vi "TestPlan - Device Mapping.vi"(7 "file path":path, 8 "error in":errorcluster, 11 "Test Type":T2 items=["Please Select", "Triaxial Shear", "Triaxial UU", "Shearbox", "Permeability", "Consolidation (Stepped Loading)/Swelling", "Saturation (Incremental)", "User Defined", "UCT", "Isotropic Consolidation", "Swelling Pressure"]) -> (0 "error out":errorcluster, 2 "Device Name":string[](array[string]), 3 "Key Name":string[](array[string]))   [LabVIEW 2019]
uses:
  Controls/Station - Tab Test Type.ctl
  Controls/Station - Test Type.ctl
  Controls/Station-state.ctl
  Controls/Station - Data Structure.ctl
  Controls/eFGV States.ctl
  Controls/Global - Device.vi
  Controls/Global - Channel.vi
  Controls/Global - Unit.vi
  <vilib>/Utility/miscctls.llb/LVRowAndColumnTypeDef.ctl
panel:
  out "ID":string
  in  "Refresh Button":bool
  out "Main Tab":enum32{"Blank", "Edit"}(tab)
  out "Sub Tab":T1
  out "Unit PPT Triaxial Shear":string caption="Cell Pressure Transducer"
  out "Unit Disp Triaxial Shear":string caption="Cell Pressure Transducer"
  out "Unit LT Triaxial Shear":string caption="Cell Pressure Transducer"
  out "Unit VC Triaxial Shear":string caption="Cell Pressure Transducer"
  out "Unit BPT Triaxial Shear":string caption="Cell Pressure Transducer"
  out "Unit CPT Triaxial Shear":string caption="Cell Pressure Transducer"
  in  "VLC Triaxial Shear":u16(ring) caption="Vertical Load Control" items=["Please Select"]
  in  "BPC Triaxial Shear":u16(ring) caption="Back Pressure Control" items=["Please Select"]
  out "Disp Triaxial Shear":sgl caption="Dispalcement" format="%.5f"
  out "PPT Triaxial Shear":sgl caption="Pore Pressure Transduser" format="%.5f"
  out "LT Triaxial Shear":sgl caption="Load Tranduser" format="%.5f"
  out "BPT Triaxial Shear":sgl caption="Back Pressure Transducer" format="%.5f"
  out "VC Triaxial Shear":sgl caption="Volume Change" format="%.5f"
  out "CPT Triaxial Shear":sgl caption="Cell Pressure Transducer" format="%.5f"
  in  "CPC Triaxial Shear":u16(ring) caption="Cell Pressure Control" items=["Please Select"]
  in  "VLC Triaxial UU":u16(ring) caption="Vertical Load Control" items=["Please Select"]
  out "CPT Triaxial UU":sgl caption="Cell Pressure" format="%.5f"
  out "VLT Triaxial UU":sgl caption="Vertical Load" format="%.5f"
  out "PPT Triaxial UU":sgl caption="Pore Pressure" format="%.5f"
  out "Disp Triaxial UU":sgl caption="Displacement" format="%.5f"
  in  "CPC Triaxial UU":u16(ring) caption="Cell Pressure Control" items=["Please Select"]
  out "Unit CPT Triaxial UU":string caption="Cell Pressure Transducer"
  out "Unit VLT Triaxial UU":string caption="Cell Pressure Transducer"
  out "Unit Disp Triaxial UU":string caption="Cell Pressure Transducer"
  out "Unit PPT Triaxial UU":string caption="Cell Pressure Transducer"
  in  "HLC Shearbox":u16(ring) caption="Horinzontal Load Control" items=["Please Select"]
  out "LT Shearbox":sgl caption="Vertical Load Tranducer" format="%.5f"
  out "Disp Shearbox":sgl caption="Vertical Dispalcement" format="%.5f"
  out "H Dis Shearbox":sgl caption="Horizontal Dispalcement" format="%.5f"
  out "HLT Shearbox":sgl caption="Horinzontal Load Tranducer" format="%.5f"
  in  "VLC Shearbox":u16(ring) caption="Vertical Load Control" items=["Please Select"]
  out "Unit LT Shearbox":string caption="Cell Pressure Transducer"
  out "Unit Disp Shearbox":string caption="Cell Pressure Transducer"
  out "Unit HLT Shearbox":string caption="Cell Pressure Transducer"
  out "Unit H Dis Shearbox":string caption="Cell Pressure Transducer"
  in  "BPC2 Permeability":u16(ring) caption="Back Pressure 2 Control" items=["Please Select"]
  in  "BPC Permeability":u16(ring) caption="Back Pressure Control" items=["Please Select"]
  out "BPT2 Permeability":sgl caption="Back Pressure 2" format="%.5f"
  out "PPT Permeability":sgl caption="Pore Pressure" format="%.5f"
  out "OVC Permeability":sgl caption="Outlet Volume Change" format="%.5f"
  out "BPT Permeability":sgl caption="Back Pressure" format="%.5f"
  out "IVC Permeability":sgl caption="Inlet Volume Change" format="%.5f"
  out "CPT Permeability":sgl caption="Cell Pressure" format="%.5f"
  in  "CPC Permeability":u16(ring) caption="Cell Pressure Control" items=["Please Select"]
  out "Unit CPT Permeability":string caption="Cell Pressure Transducer"
  out "Unit BPT Permeability":string caption="Cell Pressure Transducer"
  out "Unit IVC Permeability":string caption="Cell Pressure Transducer"
  out "Unit BPT2 Permeability":string caption="Cell Pressure Transducer"
  out "Unit OVC Permeability":string caption="Cell Pressure Transducer"
  out "Unit PPT Permeability":string caption="Cell Pressure Transducer"
  out "Disp Consolidation":sgl caption="Dispalcement"
  out "LT Consolidation":sgl caption="Load Tranducer"
  in  "VLC Consolidation":u16(ring) caption="Vertical Load  Control" items=["Please Select"]
  out "Unit LT Consolidation":string caption="Cell Pressure Transducer"
  out "Unit Disp Consolidation":string caption="Cell Pressure Transducer"
  out "CPT Saturation":sgl caption="Cell Pressure Transducer" format="%.5f"
  out "VC Saturation":sgl caption="Volume Change" format="%.5f"
  out "BPT Saturation":sgl caption="Back Pressure Transducer" format="%.5f"
  out "PPT Saturation":sgl caption="Pore pressure Tranduser" format="%.5f"
  in  "CPC Saturation":u16(ring) caption="Cell Pressure Control" items=["Please Select"]
  in  "BPC Saturation":u16(ring) caption="Back Pressure Control" items=["Please Select"]
  out "Unit CPT Saturation":string caption="Cell Pressure Transducer"
  out "Unit BPT Saturation":string caption="Cell Pressure Transducer"
  out "Unit VC Saturation":string caption="Cell Pressure Transducer"
  out "Unit PPT Saturation":string caption="Cell Pressure Transducer"
  out "HD User Defined":sgl caption="Horizontal Displacement"
  out "HL User Defined":sgl caption="Horizontal Load"
  out "VD User Defined":sgl caption="Vertical Displacement"
  out "VC2 User Defined":sgl caption="Volume Change 2"
  out "VC1 User Defined":sgl caption="Volume Change 1"
  out "VL User Defined":sgl caption="Vertical Load"
  out "BPT2 User Defined":sgl caption="Back Pressure 2"
  out "PWP User Defined":sgl caption="Pore Water Pressure"
  out "BPT User Defined":sgl caption="Back Pressure"
  out "CPT User Defined":sgl caption="Cell Pressure"
  in  "HLC User Defined":u16(ring) caption="Horizontal Load Control" items=["Please Select"]
  in  "VLC User Defined":u16(ring) caption="Vertical Load Control" items=["Please Select"]
  in  "BPC2 User Defined":u16(ring) caption="Back Pressure 2 Control" items=["Please Select"]
  in  "BPC User Defined":u16(ring) caption="Back Pressure Control" items=["Please Select"]
  in  "CPC User Defined":u16(ring) caption="Cell Pressure Control" items=["Please Select"]
  out "Unit CPT User Defined":string caption="Cell Pressure Transducer"
  out "Unit BPT User Defined":string caption="Cell Pressure Transducer"
  out "Unit VC1 User Defined":string caption="Cell Pressure Transducer"
  out "Unit PWP User Defined":string caption="Cell Pressure Transducer"
  out "Unit BPT2 User Defined":string caption="Cell Pressure Transducer"
  out "Unit VC2 User Defined":string caption="Cell Pressure Transducer"
  out "Unit HD User Defined":string caption="Cell Pressure Transducer"
  out "Unit HL User Defined":string caption="Cell Pressure Transducer"
  out "Unit VD User Defined":string caption="Cell Pressure Transducer"
  out "Unit VL User Defined":string caption="Cell Pressure Transducer"
  in  "save edit":bool
  in  "DELETE STATION":bool
  in  "Table":i32(listbox)
  in  "OK":bool
  in  "CREATE NEW STATION":bool
  # "Live Reading"
  # "Live Reading"
  # "Live Reading"
  # "Live Reading"
  # "Live Reading"
  # "Live Reading"
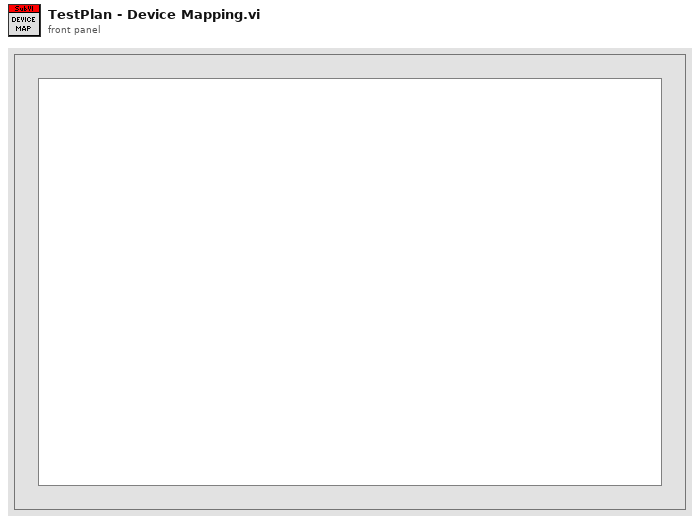
[diagram p1: front panel]
types:
  T1 = typedef "Station - Tab Test Type.ctl" = enum32{"Please Select", "Triaxial Shear", "Triaxial UU", "Shearbox", "Permeability", "Consolidation", "Saturation", "User Defined", "UCT", "Isotropic Consolidation"}
  T2 = typedef "Station - Test Type.ctl" = u16
  T3 = typedef "Station-state.ctl" = enum16{"Init", "Read Config", "Idle", "Delete", "Upload", "save edit", "update stationid", "Close", "Read sensor", "Exit"}
  T4 = typedef "eFGV States.ctl" = enum16{"Init", "Read", "Write", "Exit"}
  T5 = typedef "Station - Data Structure.ctl" = cluster{"Table station":string[][], "Station Name":string, "EditRow":i32, "Station ID":string}
  T6 = cluster{"TestPlan Section":string, "Key Value":string[]}[]
  T7 = cluster{"TestPlan Section":string, "Key Value":string[]}
  T8 = typedef "UDP - Event.ctl" = u16
  T9 = typedef "UDP - Status.ctl" = u16
  T10 = cluster{"Channels":cluster{"Ch1":sgl, "Ch2":sgl, "Ch3":sgl, "Ch4":sgl, "Ch5":sgl, "Ch6":sgl, "Ch7":sgl, "Ch8":sgl, "Ch9":sgl, "Ch10":sgl, "Ch11":sgl, "Ch12":sgl, "Ch13":sgl, "Ch14":sgl, "Ch15":sgl, "Ch16":sgl}, "Event":T8, "Status":T9, "IP":string}[]
  T11 = cluster{"Name":string[], "Unit":string[], "Decimal Point":u8[], "Ch Log":u8[], "H Alarm":u8[], "L Alarm":u8[], "H Limit":sgl[], "L Limit":sgl[], "Filter":u8[], "Gain":u8[], "Calib Type":u32[]}[]
  T12 = cluster{"Channels":cluster{"Ch1":sgl, "Ch2":sgl, "Ch3":sgl, "Ch4":sgl, "Ch5":sgl, "Ch6":sgl, "Ch7":sgl, "Ch8":sgl, "Ch9":sgl, "Ch10":sgl, "Ch11":sgl, "Ch12":sgl, "Ch13":sgl, "Ch14":sgl, "Ch15":sgl, "Ch16":sgl}, "Event":T8, "Status":T9, "IP":string}
  T13 = cluster{"Name":string[], "Unit":string[], "Decimal Point":u8[], "Ch Log":u8[], "H Alarm":u8[], "L Alarm":u8[], "H Limit":sgl[], "L Limit":sgl[], "Filter":u8[], "Gain":u8[], "Calib Type":u32[]}
  T14 = cluster{"Station Name":string, "Key Value":string[], "Key Names":string[]}[]
  T15 = cluster{"Station Name":string, "Key Value":string[], "Key Names":string[]}
  T16 = typedef "LVRowAndColumnTypeDef.ctl" = cluster{"Row":i32, "Column":i32}
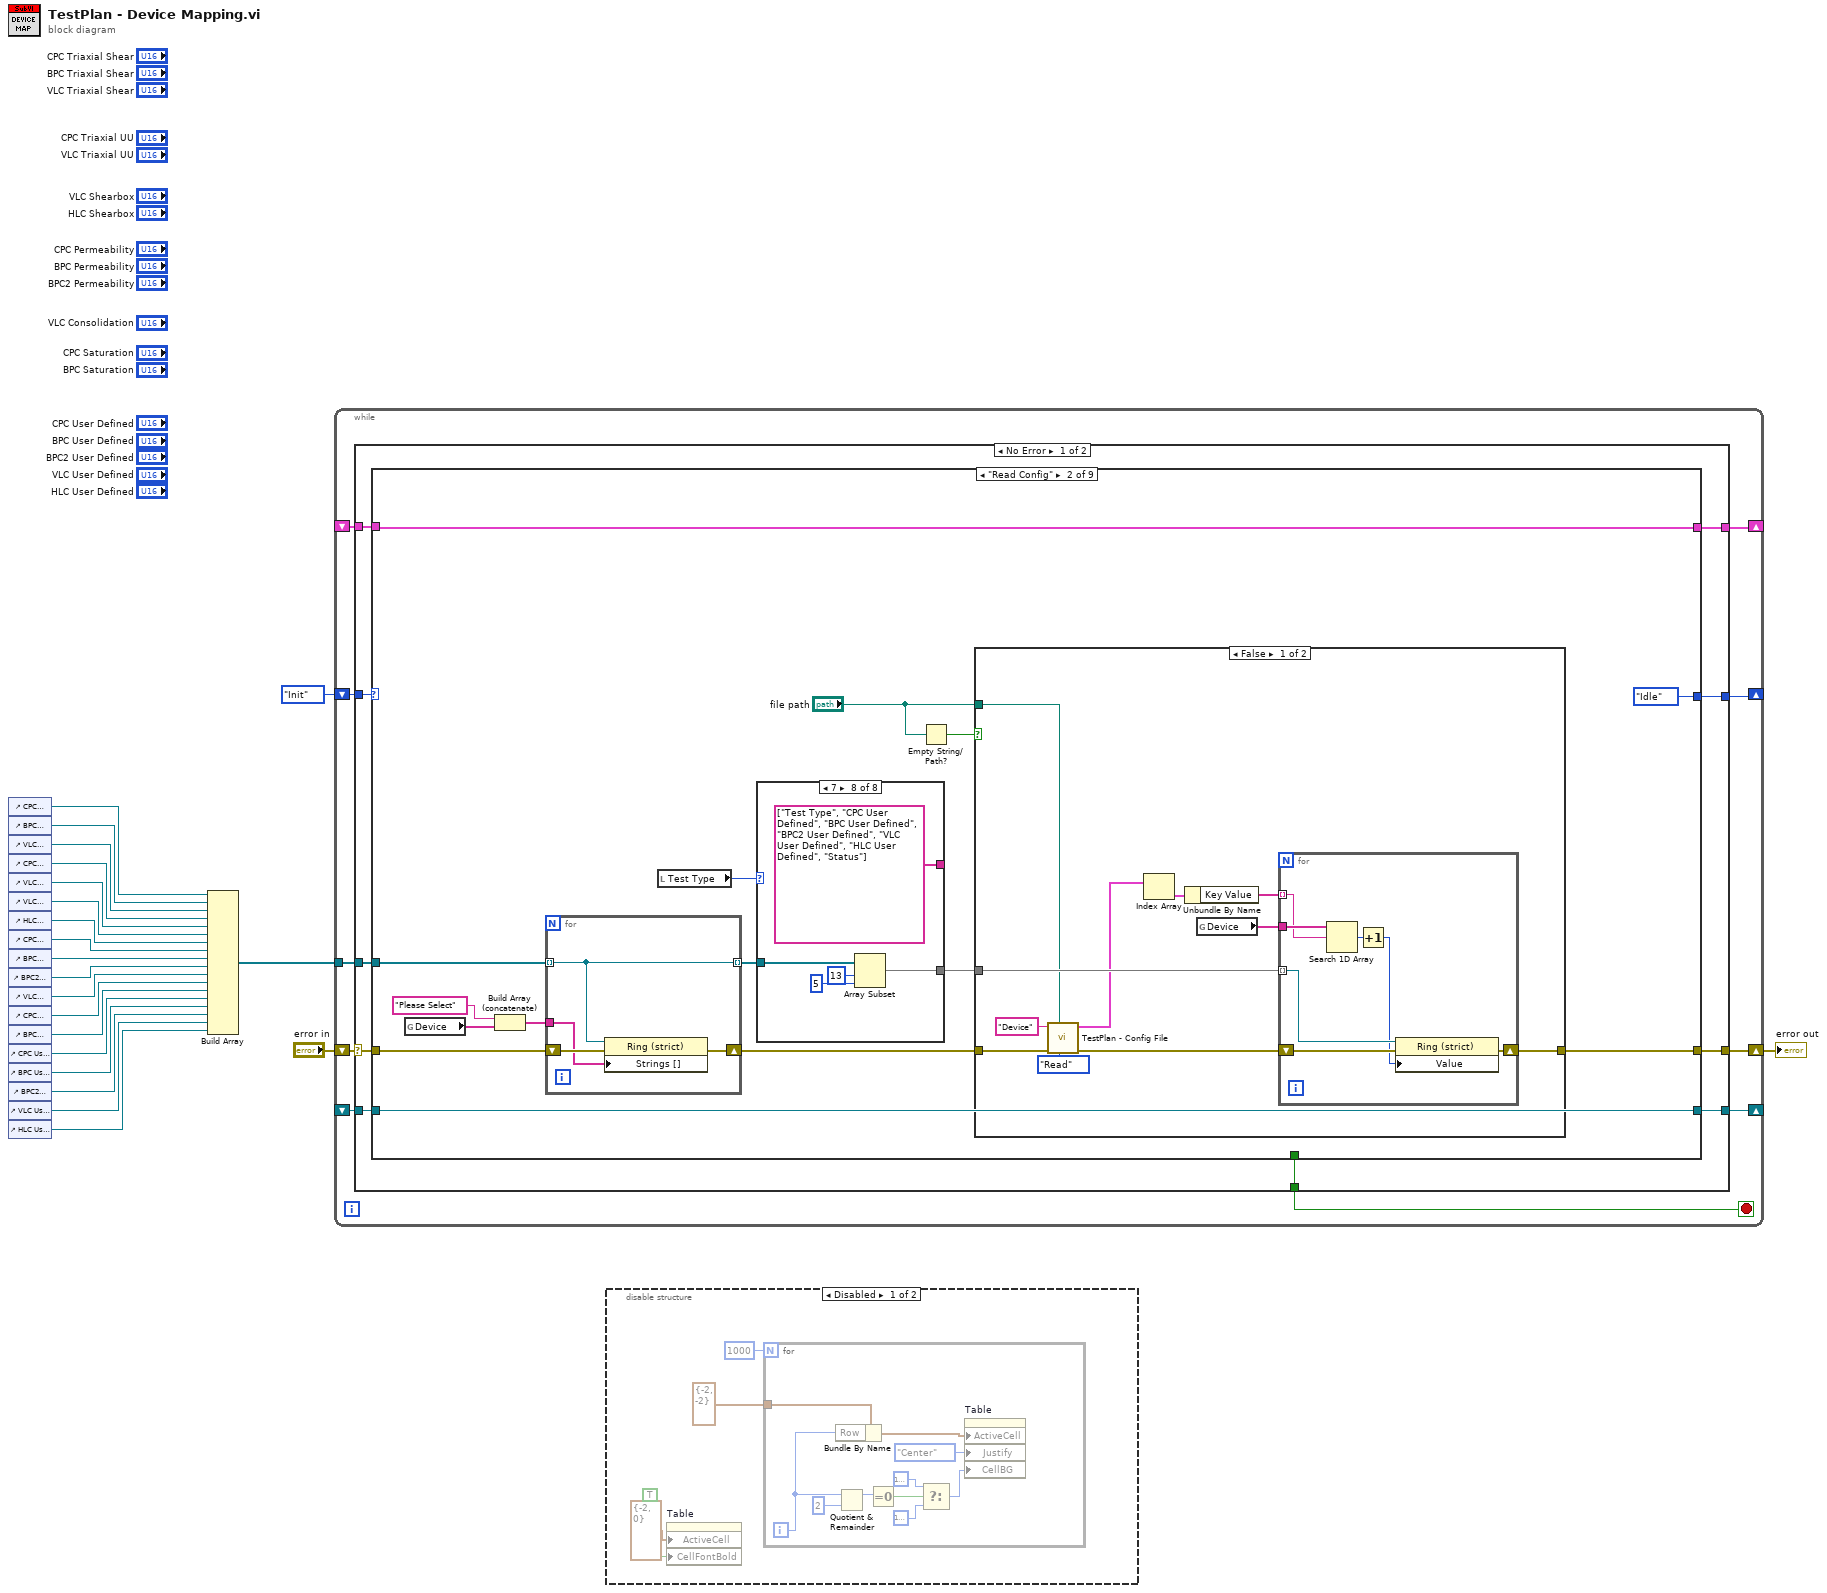
[diagram p0: block diagram]
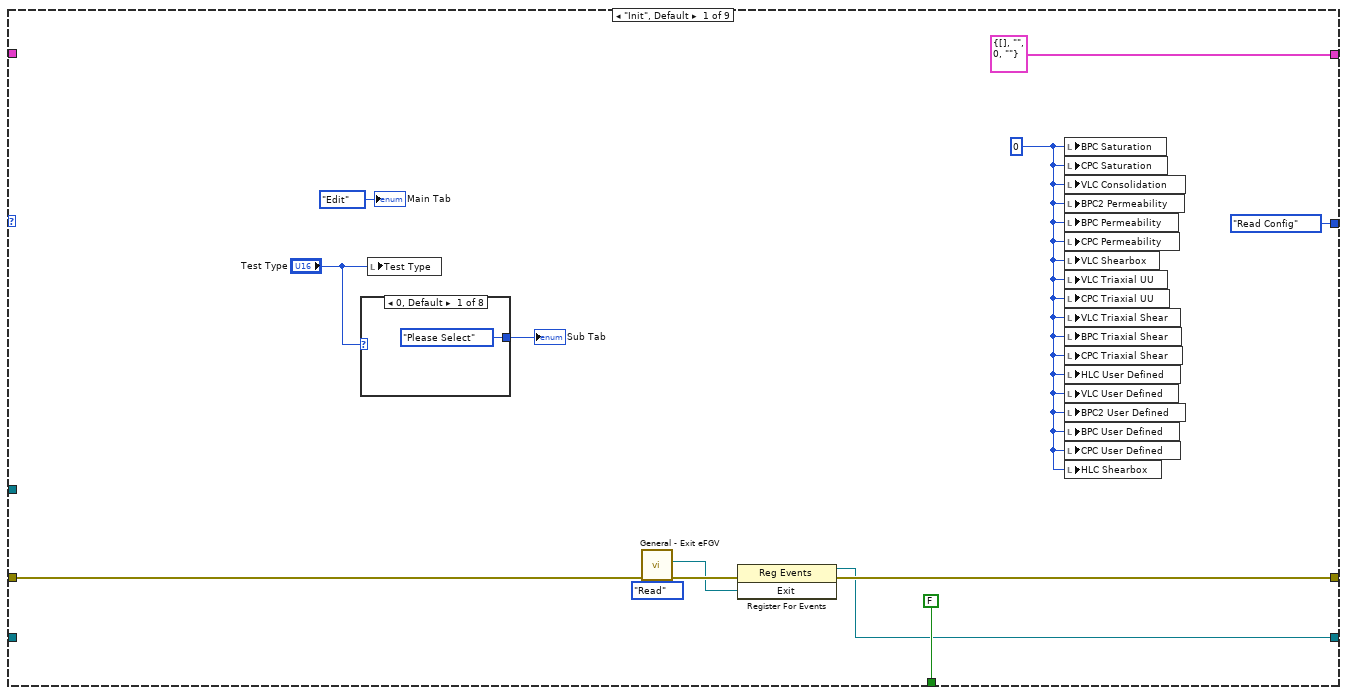
[diagram p2: hidden frame]
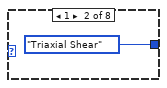
[diagram p3: hidden frame]
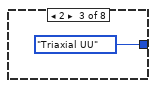
[diagram p4: hidden frame]
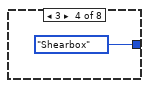
[diagram p5: hidden frame]
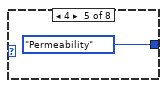
[diagram p6: hidden frame]
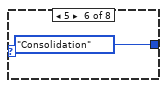
[diagram p7: hidden frame]
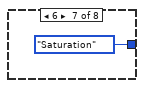
[diagram p8: hidden frame]
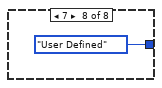
[diagram p9: hidden frame]
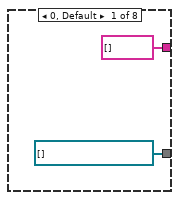
[diagram p11: hidden frame]
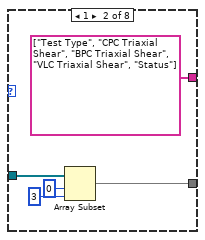
[diagram p12: hidden frame]
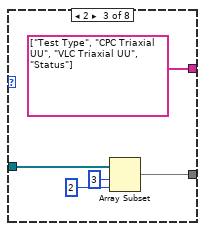
[diagram p13: hidden frame]
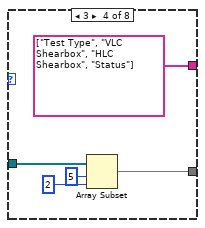
[diagram p14: hidden frame]
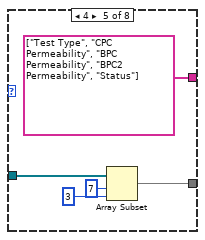
[diagram p15: hidden frame]
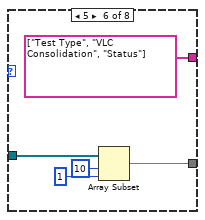
[diagram p16: hidden frame]
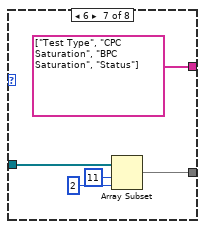
[diagram p17: hidden frame]
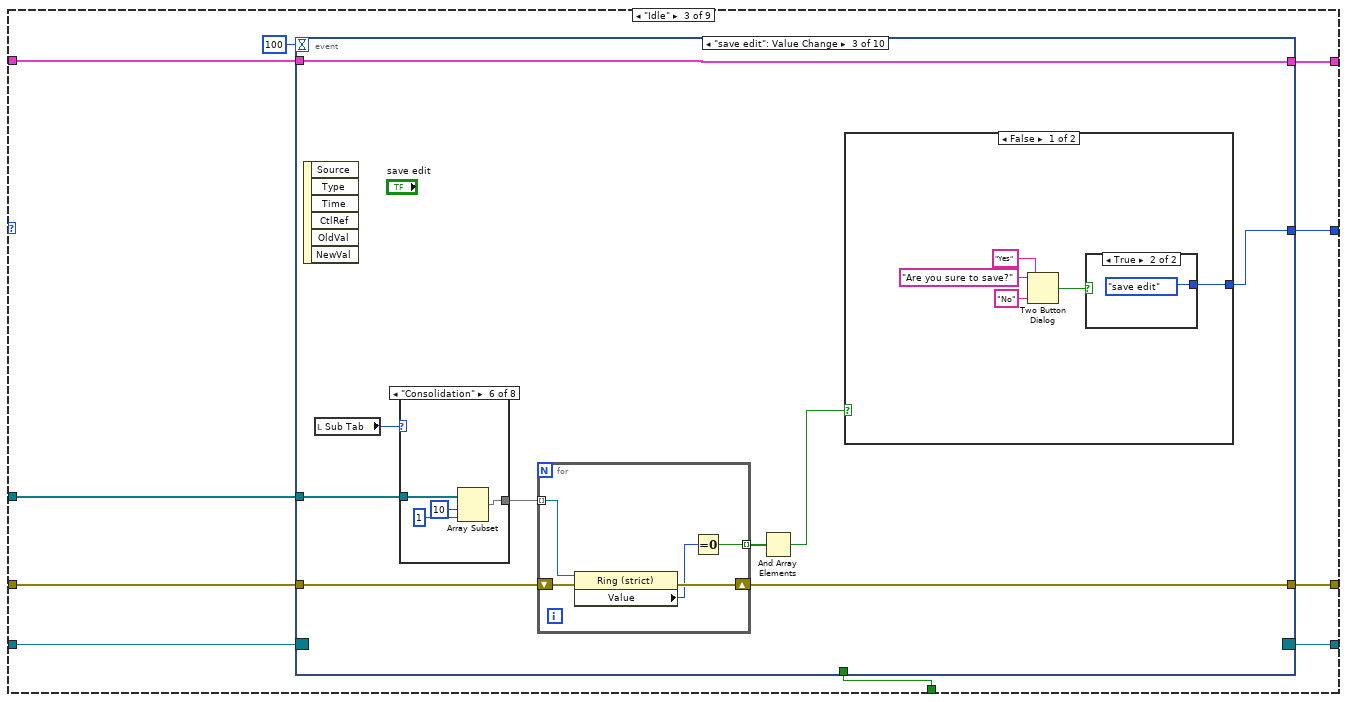
[diagram p18: hidden frame]
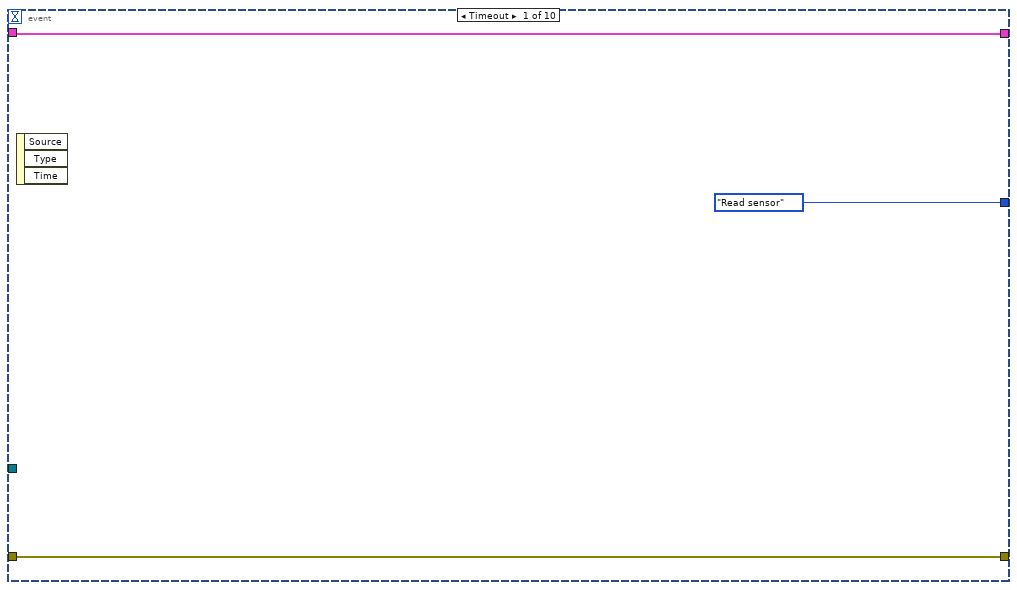
[diagram p19: hidden frame]
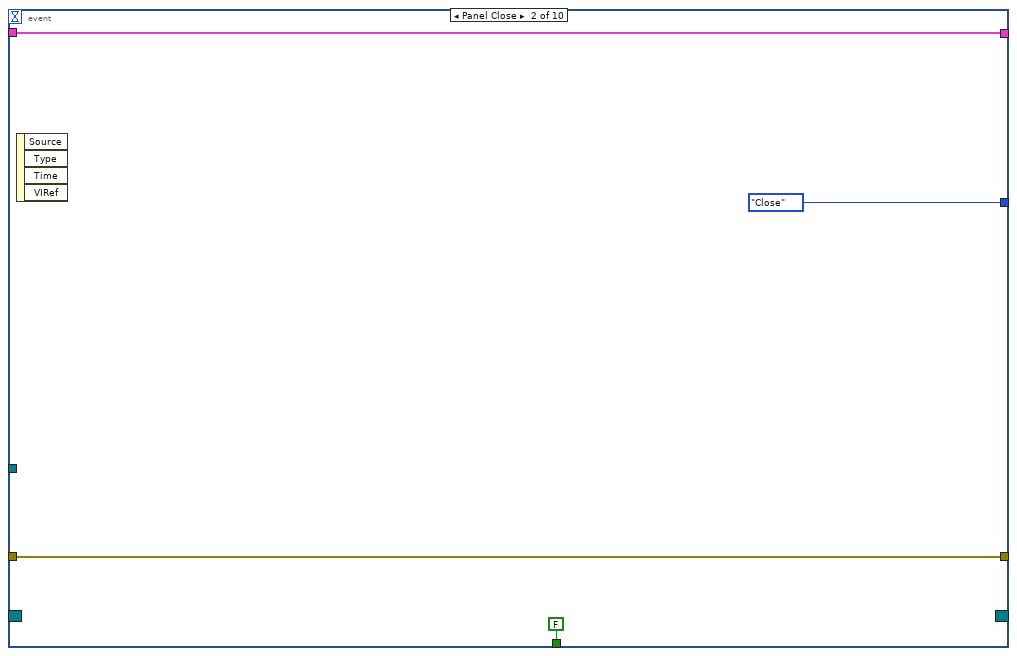
[diagram p20: hidden frame]
diagram:
  n1 = control-ref of="CPC Triaxial Shear"() -> (w19:refnum<vi>)
  n2 = control-ref of="BPC Triaxial Shear"() -> (w18:refnum<vi>)
  n3 = control-ref of="VLC Triaxial Shear"() -> (w17:refnum<vi>)
  n4 = control-ref of="CPC Triaxial UU"() -> (w16:refnum<vi>)
  n5 = control-ref of="VLC Triaxial UU"() -> (w15:refnum<vi>)
  n6 = control-ref of="VLC Shearbox"() -> (w14:refnum<vi>)
  n7 = control-ref of="HLC Shearbox"() -> (w13:refnum<vi>)
  n8 = control-ref of="CPC Permeability"() -> (w12:refnum<vi>)
  n9 = control-ref of="BPC Permeability"() -> (w11:refnum<vi>)
  n10 = control-ref of="BPC2 Permeability"() -> (w10:refnum<vi>)
  n11 = control-ref of="VLC Consolidation"() -> (w9:refnum<vi>)
  n12 = control-ref of="CPC Saturation"() -> (w8:refnum<vi>)
  n13 = control-ref of="BPC Saturation"() -> (w7:refnum<vi>)
  n14 = control-ref of="CPC User Defined"() -> (w6:refnum<vi>)
  n15 = control-ref of="BPC User Defined"() -> (w5:refnum<vi>)
  n16 = control-ref of="BPC2 User Defined"() -> (w4:refnum<vi>)
  n17 = control-ref of="VLC User Defined"() -> (w3:refnum<vi>)
  n18 = control-ref of="HLC User Defined"() -> (w2:refnum<vi>)
  n19 = Build Array(w19, w18, w17, w16, w15, w14, w13, w12, w11, w10, w9, w8, w7, w6, w5, w4, w3, w2) -> (w1:refnum<vi>[])
  n20 = while {
    shift-right: [w31] -> w21
    shift-left: "error in" -> [w32]
    shift-right: [w29] -> _
    shift-left: Station-state."Init" -> [w30]
    shift-right: [w27] -> _
    shift-left: _ -> [w26]
    shift-right: [w25] -> _
    shift-left: _ -> [w24]
    tunnel: w1 -> [w23]
    stop <- w28 stop-if-true
    n21 = case shown="No Error" w32 {
      selector: w32 -> [w41 w699]
      tunnel: [w40 w700] -> w31
      tunnel: w30 -> [w42 _]
      tunnel: [w39 Station-state."Idle"] -> w29
      tunnel: [w38 _] -> w28
      tunnel: [w37 w709] -> w27
      tunnel: w26 -> [w36 w709]
      tunnel: [w35 w707] -> w25
      tunnel: w24 -> [w34 w707]
      tunnel: w23 -> [w33 _]
      frame No Error {
        n22 = case shown="\"Read Config\"" w42 {
          tunnel: w41 -> [w43 w74 w148 w274 w553 w585 w641 w691 w692]
          tunnel: [w52 w70 w147 w273 w554 w570 w637 w688 w693] -> w40
          tunnel: [Station-state."Read Config" Station-state."Idle" w145 Station-state."Idle" Station-state."Read Config" Station-state."Idle" Station-state."Exit" Station-state."Idle" Station-state."Exit"] -> w39
          tunnel: [FALSE _ w146 _ _ _ _ _ TRUE] -> w38
          tunnel: [T5 {"Table station"=[], "Station Name"="", "EditRow"=0, "Station ID"=""} w71 w143 w279 w558 w562 w638 w690 w698] -> w37
          tunnel: w36 -> [_ w71 w144 w279 w558 w561 w638 w690 w698]
          tunnel: [w50 w77 w141 w278 w557 w590 w643 w686 w697] -> w35
          tunnel: w34 -> [_ w77 w142 w278 w557 w590 w643 w686 w697]
          tunnel: w33 -> [_ w73 w139 w271 _ w567 w640 _ _]
          frame "Init", Default {
            w46 = 0
            n23 = case shown="0, Default" "Test Type" {
              tunnel: [Station_-_Tab_Test_Type."Please Select" ("Sub Tab") Station_-_Tab_Test_Type."Triaxial Shear" ("Sub Tab") Station_-_Tab_Test_Type."Triaxial UU" ("Sub Tab") Station_-_Tab_Test_Type."Shearbox" ("Sub Tab") Station_-_Tab_Test_Type."Permeability" ("Sub Tab") Station_-_Tab_Test_Type."Consolidation" ("Sub Tab") Station_-_Tab_Test_Type."Saturation" ("Sub Tab") Station_-_Tab_Test_Type."User Defined" ("Sub Tab")] -> w44
              frame 0, Default {
              }
              frame 1 {
              }
              frame 2 {
              }
              frame 3 {
              }
              frame 4 {
              }
              frame 5 {
              }
              frame 6 {
              }
              frame 7 {
              }
            }
            "Sub Tab" <- w44
            n24 = local write "Test Type"("Test Type") -> ()
            n25 = call "General - Exit eFGV.vi"("eFGV States"=eFGV_States."Read", "error in (no error)"=w43) -> ("error out"=w53:errorcluster, "Exit"=w51:refnum<user-event>)  [unwired: 7 in, 1 out]
            n26 = register-events(error in=w53, w51) -> (reference out=w50:refnum<event-registration>, error out=w52:errorcluster)  [unwired: 1 in]
            n27 = local write "BPC Saturation"(w46) -> ()
            n28 = local write "CPC Saturation"(w46) -> ()
            n29 = local write "VLC Consolidation"(w46) -> ()
            n30 = local write "BPC2 Permeability"(w46) -> ()
            n31 = local write "BPC Permeability"(w46) -> ()
            n32 = local write "CPC Permeability"(w46) -> ()
            n33 = local write "VLC Shearbox"(w46) -> ()
            n34 = local write "VLC Triaxial UU"(w46) -> ()
            n35 = local write "CPC Triaxial UU"(w46) -> ()
            n36 = local write "VLC Triaxial Shear"(w46) -> ()
            n37 = local write "BPC Triaxial Shear"(w46) -> ()
            n38 = local write "CPC Triaxial Shear"(w46) -> ()
            n39 = local write "HLC User Defined"(w46) -> ()
            n40 = local write "VLC User Defined"(w46) -> ()
            n41 = local write "BPC2 User Defined"(w46) -> ()
            n42 = local write "BPC User Defined"(w46) -> ()
            n43 = local write "CPC User Defined"(w46) -> ()
            n44 = local write "HLC Shearbox"(w46) -> ()
            "Main Tab" <- enum32{"Blank", "Edit"}."Edit" ("Main Tab")
          }
          frame "Read Config" {
            n45 = global read "Global - Device.vi" "Device"() -> (w72:string[])
            n46 = Build Array (concatenate)("Please Select", w72) -> (w75:string[])
            n47 = for {
              shift-right: [w137] -> w66
              shift-left: w74 -> [w138]
              tunnel: w73 -> [w135] mode=indexing
              tunnel: w75 -> [w136]
              tunnel: [w135] -> w69 mode=indexing
              n48 = property class="Ring (strict)"(reference=w135, error in=w138, "Strings []"=w136) -> (error out=w137:errorcluster)  [unwired: 1 out]
            }
            n49 = local read "Test Type"() -> (w68:T2)
            n50 = case shown="7" w68 {
              tunnel: [string[] [] string[] ["Test Type", "CPC Triaxial Shear", "BPC Triaxial Shear", "VLC Triaxial Shear", "Status"] string[] ["Test Type", "CPC Triaxial UU", "VLC Triaxial UU", "Status"] string[] ["Test Type", "VLC Shearbox", "HLC Shearbox", "Status"] string[] ["Test Type", "CPC Permeability", "BPC Permeability", "BPC2 Permeability", "Status"] string[] ["Test Type", "VLC Consolidation", "Status"] string[] ["Test Type", "CPC Saturation", "BPC Saturation", "Status"] string[] ["Test Type", "CPC User Defined", "BPC User Defined", "BPC2 User Defined", "VLC User Defined", "HLC User Defined", "Status"]] -> _
              tunnel: w69 -> [_ w103 w106 w111 w116 w121 w126 w131]
              tunnel: [refnum<vi>[] [] w100 w105 w110 w115 w120 w125 w130] -> w67
              frame 0, Default {
              }
              frame 1 {
                n51 = Array Subset(array=w103, index=0, length=3) -> (w100:refnum<vi>[])
              }
              frame 2 {
                n52 = Array Subset(array=w106, index=3, length=2) -> (w105:refnum<vi>[])
              }
              frame 3 {
                n53 = Array Subset(array=w111, index=5, length=2) -> (w110:refnum<vi>[])
              }
              frame 4 {
                n54 = Array Subset(array=w116, index=7, length=3) -> (w115:refnum<vi>[])
              }
              frame 5 {
                n55 = Array Subset(array=w121, index=10, length=1) -> (w120:refnum<vi>[])
              }
              frame 6 {
                n56 = Array Subset(array=w126, index=11, length=2) -> (w125:refnum<vi>[])
              }
              frame 7 {
                n57 = Array Subset(array=w131, index=13, length=5) -> (w130:refnum<vi>[])
              }
            }
            n58 = Empty String/Path?(string/path="file path") -> (empty?=w64:bool)
            n59 = case shown="False" w64 {
              tunnel: [w88 w97] -> w70
              tunnel: w67 -> [w87 _]
              tunnel: w66 -> [w85 w97]
              tunnel: "file path" -> [w79 _]
              frame False {
                n60 = call "TestPlan - Config File.vi"("Action"=enum16{"Write", "Read", "Read All", "Remove"}."Read", "file path"=w79, "error in (no error)"=w85, "TestPlan Section"="Device") -> ("error out"=w84:errorcluster, "Value Out"=w83:T6)  [unwired: 5 in, 1 out]
                n61 = Index Array(array=w83) -> (element=w81:T7)  [unwired: 1 in]
                n62 = Unbundle By Name(w81) -> ("Key Value"=w80:string[])
                n63 = global read "Global - Device.vi" "Device"() -> (w89:string[])
                n64 = for {
                  tunnel: w80 -> [w95] mode=indexing
                  tunnel: w89 -> [w96]
                  shift-right: [w93] -> w88
                  shift-left: w84 -> [w94]
                  tunnel: w87 -> [w92] mode=indexing
                  n65 = Search 1D Array(1D array=w96, element=w95) -> (index of element=w91:i32)  [unwired: 1 in]
                  n66 = Increment(x=w91) -> (x+1=w90:i32)
                  n67 = property class="Ring (strict)"(reference=w92, error in=w94, "Value"=w90) -> (error out=w93:errorcluster)  [unwired: 1 out]
                }
              }
              frame True {
              }
            }
          }
          frame "Idle" {
            n68 = event shown="[2] \"save edit\": Value Change" {
              selector: w142 -> [_ _ _ _ _ _ _ _ _ _]
              dyn-events: [_ _ _ _ _ _ _ _ _ _] -> w141
              timeout: 100 -> [_ _ _ _ _ _ _ _ _ _]
              tunnel: w148 -> [w149 w155 w159 w209 w229 w232 w238 w247 w250 w252]
              tunnel: [w149 w155 w156 w209 w229 w232 w237 w247 w250 w253] -> w147
              tunnel: [_ FALSE _ _ _ _ _ _ FALSE _] -> w146
              tunnel: [Station-state."Read sensor" Station-state."Close" w163 Station-state."Idle" w225 Station-state."Read Config" w234 Station-state."Exit" Station-state."Close" w257] -> w145
              tunnel: w144 -> [w151 w154 w164 w211 w221 w231 w239 w246 w249 w254]
              tunnel: [w151 w154 w164 w211 w221 w231 w239 w246 w249 w255] -> w143
              tunnel: w139 -> [_ _ w162 _ _ _ _ _ _ _]
              event Timeout {
                n69 = event-data() -> ()  [unwired: 1 in, 3 out]
              }
              event Panel Close {
                n70 = event-data() -> ()  [unwired: 1 in, 4 out]
              }
              event "save edit": Value Change {
                n71 = event-data() -> ()  [unwired: 1 in, 6 out]
                n72 = local read "Sub Tab"() -> (w161:T1)
                n73 = case shown="\"Consolidation\"" w161 {
                  tunnel: w162 -> [_ w183 w185 w189 w193 w197 w201 w205]
                  tunnel: [_ w180 w184 w188 w192 w196 w200 w204] -> w160
                  frame "Please Select", Default {
                  }
                  frame "Triaxial Shear" {
                    n74 = Array Subset(array=w183, index=0, length=3) -> (w180:refnum<vi>[])
                  }
                  frame "Triaxial UU" {
                    n75 = Array Subset(array=w185, index=3, length=2) -> (w184:refnum<vi>[])
                  }
                  frame "Shearbox" {
                    n76 = Array Subset(array=w189, index=5, length=2) -> (w188:refnum<vi>[])
                  }
                  frame "Permeability" {
                    n77 = Array Subset(array=w193, index=7, length=3) -> (w192:refnum<vi>[])
                  }
                  frame "Consolidation" {
                    n78 = Array Subset(array=w197, index=10, length=1) -> (w196:refnum<vi>[])
                  }
                  frame "Saturation" {
                    n79 = Array Subset(array=w201, index=11, length=2) -> (w200:refnum<vi>[])
                  }
                  frame "User Defined" {
                    n80 = Array Subset(array=w205, index=13, length=5) -> (w204:refnum<vi>[])
                  }
                }
                n81 = for {
                  tunnel: w160 -> [w177] mode=indexing
                  shift-right: [w178] -> w156
                  shift-left: w159 -> [w179]
                  tunnel: [w175] -> w158 mode=indexing
                  n82 = property class="Ring (strict)"(reference=w177, error in=w179) -> (error out=w178:errorcluster, "Value"=w176:u16)  [unwired: 1 out]
                  n83 = Equal To 0?(x=w176) -> (x = 0?=w175:bool)
                }
                n84 = And Array Elements(Boolean array=w158) -> (logical AND=w157:bool)
                n85 = case shown="False" w157 {
                  tunnel: [w169 Station-state."Idle"] -> w163
                  frame False {
                    n86 = Two Button Dialog(message="Are you sure to save?", 1:"No" ("F button name (\"Cancel\")"), 2:"Yes" ("T button name (\"OK\")")) -> (T button?=w168:bool)
                    n87 = case shown="True" w168 {
                      tunnel: [Station-state."Idle" Station-state."save edit"] -> w169
                      frame False {
                      }
                      frame True {
                      }
                    }
                  }
                  frame True {
                    n88 = One Button Dialog(message="Please Select Device", button name ("OK")="OK") -> ()  [unwired: 1 out]
                  }
                }
              }
              event Value Change {
                n89 = event-data() -> ("NewVal"=w210:T2)  [unwired: 1 in, 5 out]
                n90 = case shown="0, Default" w210 {
                  tunnel: [Station_-_Tab_Test_Type."Please Select" ("Sub Tab") Station_-_Tab_Test_Type."Triaxial Shear" ("Sub Tab") Station_-_Tab_Test_Type."Triaxial UU" ("Sub Tab") Station_-_Tab_Test_Type."Shearbox" ("Sub Tab") Station_-_Tab_Test_Type."Permeability" ("Sub Tab") Station_-_Tab_Test_Type."Consolidation" ("Sub Tab") Station_-_Tab_Test_Type."Saturation" ("Sub Tab") Station_-_Tab_Test_Type."User Defined" ("Sub Tab")] -> w208
                  frame 0, Default {
                  }
                  frame 1 {
                  }
                  frame 2 {
                  }
                  frame 3 {
                  }
                  frame 4 {
                  }
                  frame 5 {
                  }
                  frame 6 {
                  }
                  frame 7 {
                  }
                }
                n91 = local write "Sub Tab"(w208) -> ()
              }
              event "DELETE STATION": Value Change {
                n92 = event-data() -> ()  [unwired: 1 in, 6 out]
                n93 = Two Button Dialog(message="Are you sure to delete?", 1:"No" ("F button name (\"Cancel\")"), 2:"Yes" ("T button name (\"OK\")")) -> (T button?=w222:bool)
                n94 = Select(t=Station-state."Delete", s=w222, f=Station-state."Idle") -> (s? t:f=w225:T3)
              }
              event "Refresh Button": Value Change {
                n95 = event-data() -> ()  [unwired: 1 in, 6 out]
              }
              event "CREATE NEW STATION": Value Change {
                n96 = event-data() -> ()  [unwired: 1 in, 6 out]
                n97 = disable-structure shown="Enabled" {
                  disable-tunnel: w238 -> [w242 w243]
                  disable-tunnel: [w241 w243] -> w237
                  disable-tunnel: [w240 TRUE ("ForceClose")] -> w236
                  frame Disabled {
                    n98 = call "Station - Create New Station (SubVI).vi"("error constant"=w242) -> ("error out"=w241:errorcluster, "ForceClose"=w240:bool)  [unwired: 7 in, 2 out]
                  }
                  frame Enabled {
                  }
                }
                n99 = Select(t=Station-state."Idle", s=w236, f=Station-state."Read Config") -> (s? t:f=w234:T3)
              }
              event User Event {
                n100 = event-data() -> ()  [unwired: 1 in, 5 out]
              }
              event "OK": Value Change {
                n101 = event-data() -> ()  [unwired: 1 in, 6 out]
              }
              event "Table": Mouse Down {
                n102 = event-data() -> ("Mods.Double Click"=w256:bool)  [unwired: 1 in]
                n103 = case shown="True" w256 {
                  tunnel: [Station-state."Idle" Station-state."Upload"] -> w257
                  tunnel: w254 -> [w260 w264]
                  tunnel: [w260 w268] -> w255
                  tunnel: w252 -> [w258 w267]
                  tunnel: [w258 w267] -> w253
                  frame False {
                  }
                  frame True {
                    n104 = Unbundle By Name(w264) -> ("Table station"=w266:string[][])
                    n105 = Index Array(array=w266, index (row)="Table", index (col)=1 ("disabled index (col)")) -> (element=w261:string)
                    n106 = Bundle By Name(cluster=w264, "Station Name"=w261, "EditRow"="Table") -> (w268:T5)
                    n107 = local write "Main Tab"(enum32{"Blank", "Edit"}."Edit" ("Main Tab")) -> ()
                  }
                }
              }
            }
          }
          frame "Read sensor" {
            n108 = local read "Sub Tab"() -> (w272:T1)
            n109 = call "Station - Search Serial Number by Device Name.vi"("error in (no error)"=w274, "Array in"=w271) -> ("error out"=w276:errorcluster, "Index"=w270:i32[])  [unwired: 6 in, 2 out]
            n110 = case shown="\"Please Select\", Default" w272 {
              tunnel: w270 -> [_ w527 w529 w533 w537 w541 w545 w549]
              tunnel: [i32[] [] w524 w528 w532 w536 w540 w544 w548] -> w275
              frame "Please Select", Default {
              }
              frame "Triaxial Shear" {
                n111 = Array Subset(array=w527, index=0, length=3) -> (w524:i32[])
              }
              frame "Triaxial UU" {
                n112 = Array Subset(array=w529, index=3, length=2) -> (w528:i32[])
              }
              frame "Shearbox" {
                n113 = Array Subset(array=w533, index=5, length=2) -> (w532:i32[])
              }
              frame "Permeability" {
                n114 = Array Subset(array=w537, index=7, length=3) -> (w536:i32[])
              }
              frame "Consolidation" {
                n115 = Array Subset(array=w541, index=10, length=1) -> (w540:i32[])
              }
              frame "Saturation" {
                n116 = Array Subset(array=w545, index=11, length=2) -> (w544:i32[])
              }
              frame "User Defined" {
                n117 = Array Subset(array=w549, index=13, length=5) -> (w548:i32[])
              }
            }
            n118 = for {
              shift-right: [w296] -> w273
              shift-left: w276 -> [w291]
              tunnel: w275 -> [w290] mode=indexing
              tunnel: w272 -> [w294]
              i -> [w295]
              n119 = global read "Global - Channel.vi" "Data"() -> (w287:T10)
              n120 = global read "Global - Unit.vi" "Unit"() -> (w286:T11)
              n121 = Index Array(array=w287, index=w290) -> (element=w289:T12)
              n122 = Index Array(array=w286, index=w290) -> (element=w288:T13)
              n123 = Unbundle By Name(w288) -> ("Unit"=w285:string[], "Decimal Point"=w282:u8[])
              n124 = Unbundle By Name(w289) -> ("Channels.Ch1"=w293:sgl, "Channels.Ch2"=w292:sgl)
              n125 = Index Array(array=w285) -> (element #1=w284:string, element #2=w283:string)  [unwired: 2 in]
              n126 = Index Array(array=w282) -> (element #1=w281:u8, element #2=w280:u8)  [unwired: 2 in]
              n127 = case shown="\"User Defined\"" w294 {
                tunnel: [w297 w306 w342 w369 w396 w432 w450 w477] -> w296
                tunnel: w291 -> [w297 w305 w341 w368 w395 w431 w449 w476]
                tunnel: w295 -> [_ w304 w340 w367 w394 w430 w448 w475]
                tunnel: w293 -> [_ w303 w339 w366 w393 w429 w447 w474]
                tunnel: w284 -> [_ w302 w337 w364 w391 w427 w445 w472]
                tunnel: w283 -> [_ w301 w336 w363 w390 w426 w444 w471]
                tunnel: w292 -> [_ w300 w338 w365 w392 w428 w446 w473]
                tunnel: w281 -> [_ w299 w335 w362 w389 w424 w442 w469]
                tunnel: w280 -> [_ w298 w334 w361 w388 w425 w443 w470]
                frame "Please Select", Default {
                }
                frame "Triaxial Shear" {
                  n128 = case shown="2" w304 {
                    tunnel: [w310 w319 w328] -> w306
                    tunnel: w305 -> [w309 w318 w327]
                    tunnel: w303 -> [w315 w324 w331]
                    tunnel: w302 -> [w314 w323 w333]
                    tunnel: w301 -> [w313 w322 w332]
                    tunnel: w300 -> [w312 w321 w330]
                    tunnel: w299 -> [w307 w316 w326]
                    tunnel: w298 -> [w308 w317 w325]
                    frame 0, Default {
                      n129 = property on="CPT Triaxial Shear" class="DigNum (strict)"(error in=w309, "Precision"=w308) -> (error out=w311:errorcluster)  [unwired: 1 in, 1 out]
                      n130 = property on="PPT Triaxial Shear" class="DigNum (strict)"(error in=w311, "Precision"=w307) -> (error out=w310:errorcluster)  [unwired: 1 in, 1 out]
                      "CPT Triaxial Shear" <- w315
                      "PPT Triaxial Shear" <- w312
                      "Unit CPT Triaxial Shear" <- w314
                      "Unit PPT Triaxial Shear" <- w313
                    }
                    frame 1 {
                      n131 = property on="BPT Triaxial Shear" class="DigNum (strict)"(error in=w318, "Precision"=w317) -> (error out=w320:errorcluster)  [unwired: 1 in, 1 out]
                      n132 = property on="VC Triaxial Shear" class="DigNum (strict)"(error in=w320, "Precision"=w316) -> (error out=w319:errorcluster)  [unwired: 1 in, 1 out]
                      "VC Triaxial Shear" <- w321
                      "BPT Triaxial Shear" <- w324
                      "Unit BPT Triaxial Shear" <- w323
                      "Unit VC Triaxial Shear" <- w322
                    }
                    frame 2 {
                      n133 = property on="LT Triaxial Shear" class="DigNum (strict)"(error in=w327, "Precision"=w325) -> (error out=w329:errorcluster)  [unwired: 1 in, 1 out]
                      n134 = property on="Disp Triaxial Shear" class="DigNum (strict)"(error in=w329, "Precision"=w326) -> (error out=w328:errorcluster)  [unwired: 1 in, 1 out]
                      "LT Triaxial Shear" <- w331
                      "Disp Triaxial Shear" <- w330
                      "Unit LT Triaxial Shear" <- w333
                      "Unit Disp Triaxial Shear" <- w332
                    }
                  }
                }
                frame "Triaxial UU" {
                  n135 = case shown="1" w340 {
                    tunnel: [w347 w357] -> w342
                    tunnel: w341 -> [w346 w356]
                    tunnel: w339 -> [w351 w360]
                    tunnel: w338 -> [w350 w359]
                    tunnel: w337 -> [w349 w352]
                    tunnel: w336 -> [w343 w353]
                    tunnel: w335 -> [w345 w355]
                    tunnel: w334 -> [w344 w354]
                    frame 0, Default {
                      n136 = property on="CPT Triaxial UU" class="DigNum (strict)"(error in=w346, "Precision"=w344) -> (error out=w348:errorcluster)  [unwired: 1 in, 1 out]
                      n137 = property on="PPT Triaxial UU" class="DigNum (strict)"(error in=w348, "Precision"=w345) -> (error out=w347:errorcluster)  [unwired: 1 in, 1 out]
                      "PPT Triaxial UU" <- w350
                      "CPT Triaxial UU" <- w351
                      "Unit CPT Triaxial UU" <- w349
                      "Unit PPT Triaxial UU" <- w343
                    }
                    frame 1 {
                      n138 = property on="VLT Triaxial UU" class="DigNum (strict)"(error in=w356, "Precision"=w354) -> (error out=w358:errorcluster)  [unwired: 1 in, 1 out]
                      n139 = property on="Disp Triaxial UU" class="DigNum (strict)"(error in=w358, "Precision"=w355) -> (error out=w357:errorcluster)  [unwired: 1 in, 1 out]
                      "Disp Triaxial UU" <- w359
                      "VLT Triaxial UU" <- w360
                      "Unit Disp Triaxial UU" <- w353
                      "Unit VLT Triaxial UU" <- w352
                    }
                  }
                }
                frame "Shearbox" {
                  n140 = case shown="0, Default" w367 {
                    tunnel: [w373 w382] -> w369
                    tunnel: w368 -> [w372 w381]
                    tunnel: w366 -> [w378 w387]
                    tunnel: w365 -> [w377 w386]
                    tunnel: w364 -> [w376 w385]
                    tunnel: w363 -> [w375 w384]
                    tunnel: w362 -> [w371 w380]
                    tunnel: w361 -> [w370 w379]
                    frame 0, Default {
                      n141 = property on="LT Shearbox" class="DigNum (strict)"(error in=w372, "Precision"=w370) -> (error out=w374:errorcluster)  [unwired: 1 in, 1 out]
                      n142 = property on="Disp Shearbox" class="DigNum (strict)"(error in=w374, "Precision"=w371) -> (error out=w373:errorcluster)  [unwired: 1 in, 1 out]
                      "LT Shearbox" <- w378
                      "Disp Shearbox" <- w377
                      "Unit Disp Shearbox" <- w375
                      "Unit LT Shearbox" <- w376
                    }
                    frame 1 {
                      n143 = property on="HLT Shearbox" class="DigNum (strict)"(error in=w381, "Precision"=w379) -> (error out=w383:errorcluster)  [unwired: 1 in, 1 out]
                      n144 = property on="H Dis Shearbox" class="DigNum (strict)"(error in=w383, "Precision"=w380) -> (error out=w382:errorcluster)  [unwired: 1 in, 1 out]
                      "HLT Shearbox" <- w387
                      "H Dis Shearbox" <- w386
                      "Unit HLT Shearbox" <- w385
                      "Unit H Dis Shearbox" <- w384
                    }
                  }
                }
                frame "Permeability" {
                  n145 = case shown="0, Default" w394 {
                    tunnel: [w400 w409 w418] -> w396
                    tunnel: w395 -> [w399 w408 w417]
                    tunnel: w393 -> [w405 w414 w423]
                    tunnel: w392 -> [w404 w413 w422]
                    tunnel: w391 -> [w403 w412 w421]
                    tunnel: w390 -> [w402 w411 w420]
                    tunnel: w389 -> [w398 w407 w415]
                    tunnel: w388 -> [w397 w406 w416]
                    frame 0, Default {
                      n146 = property on="CPT Permeability" class="DigNum (strict)"(error in=w399, "Precision"=w397) -> (error out=w401:errorcluster)  [unwired: 1 in, 1 out]
                      n147 = property on="PPT Permeability" class="DigNum (strict)"(error in=w401, "Precision"=w398) -> (error out=w400:errorcluster)  [unwired: 1 in, 1 out]
                      "CPT Permeability" <- w405
                      "PPT Permeability" <- w404
                      "Unit CPT Permeability" <- w403
                      "Unit PPT Permeability" <- w402
                    }
                    frame 1 {
                      n148 = property on="BPT Permeability" class="DigNum (strict)"(error in=w408, "Precision"=w406) -> (error out=w410:errorcluster)  [unwired: 1 in, 1 out]
                      n149 = property on="IVC Permeability" class="DigNum (strict)"(error in=w410, "Precision"=w407) -> (error out=w409:errorcluster)  [unwired: 1 in, 1 out]
                      "IVC Permeability" <- w413
                      "BPT Permeability" <- w414
                      "Unit BPT Permeability" <- w412
                      "Unit IVC Permeability" <- w411
                    }
                    frame 2 {
                      n150 = property on="BPT2 Permeability" class="DigNum (strict)"(error in=w417, "Precision"=w416) -> (error out=w419:errorcluster)  [unwired: 1 in, 1 out]
                      n151 = property on="OVC Permeability" class="DigNum (strict)"(error in=w419, "Precision"=w415) -> (error out=w418:errorcluster)  [unwired: 1 in, 1 out]
                      "OVC Permeability" <- w422
                      "BPT2 Permeability" <- w423
                      "Unit BPT2 Permeability" <- w421
                      "Unit OVC Permeability" <- w420
                    }
                  }
                }
                frame "Consolidation" {
                  n152 = case shown="0, Default" w430 {
                    tunnel: [w436] -> w432
                    tunnel: w431 -> [w435]
                    tunnel: w429 -> [w441]
                    tunnel: w428 -> [w440]
                    tunnel: w427 -> [w439]
                    tunnel: w426 -> [w438]
                    tunnel: w425 -> [w434]
                    tunnel: w424 -> [w433]
                    frame 0, Default {
                      n153 = property on="LT Consolidation" class="DigNum (strict)"(error in=w435, "Precision"=w434) -> (error out=w437:errorcluster)  [unwired: 1 in, 1 out]
                      n154 = property on="Disp Consolidation" class="DigNum (strict)"(error in=w437, "Precision"=w433) -> (error out=w436:errorcluster)  [unwired: 1 in, 1 out]
                      "LT Consolidation" <- w441
                      "Disp Consolidation" <- w440
                      "Unit LT Consolidation" <- w439
                      "Unit Disp Consolidation" <- w438
                    }
                  }
                }
                frame "Saturation" {
                  n155 = case shown="0, Default" w448 {
                    tunnel: [w454 w463] -> w450
                    tunnel: w449 -> [w453 w462]
                    tunnel: w447 -> [w459 w468]
                    tunnel: w446 -> [w458 w467]
                    tunnel: w445 -> [w457 w466]
                    tunnel: w444 -> [w456 w465]
                    tunnel: w443 -> [w452 w461]
                    tunnel: w442 -> [w451 w460]
                    frame 0, Default {
                      n156 = property on="CPT Saturation" class="DigNum (strict)"(error in=w453, "Precision"=w452) -> (error out=w455:errorcluster)  [unwired: 1 in, 1 out]
                      n157 = property on="PPT Saturation" class="DigNum (strict)"(error in=w455, "Precision"=w451) -> (error out=w454:errorcluster)  [unwired: 1 in, 1 out]
                      "CPT Saturation" <- w459
                      "PPT Saturation" <- w458
                      "Unit CPT Saturation" <- w457
                      "Unit PPT Saturation" <- w456
                    }
                    frame 1 {
                      n158 = property on="BPT Saturation" class="DigNum (strict)"(error in=w462, "Precision"=w461) -> (error out=w464:errorcluster)  [unwired: 1 in, 1 out]
                      n159 = property on="VC Saturation" class="DigNum (strict)"(error in=w464, "Precision"=w460) -> (error out=w463:errorcluster)  [unwired: 1 in, 1 out]
                      "BPT Saturation" <- w468
                      "VC Saturation" <- w467
                      "Unit BPT Saturation" <- w466
                      "Unit VC Saturation" <- w465
                    }
                  }
                }
                frame "User Defined" {
                  n160 = case shown="0, Default" w475 {
                    tunnel: [w481 w490 w499 w508 w517] -> w477
                    tunnel: w476 -> [w480 w489 w498 w507 w516]
                    tunnel: w474 -> [w486 w495 w504 w513 w522]
                    tunnel: w473 -> [w485 w494 w503 w512 w521]
                    tunnel: w472 -> [w484 w493 w502 w511 w520]
                    tunnel: w471 -> [w483 w492 w501 w510 w519]
                    tunnel: w470 -> [w479 w488 w497 w505 w515]
                    tunnel: w469 -> [w478 w487 w496 w506 w514]
                    frame 0, Default {
                      n161 = property on="CPT User Defined" class="DigNum (strict)"(error in=w480, "Precision"=w479) -> (error out=w482:errorcluster)  [unwired: 1 in, 1 out]
                      n162 = property on="PWP User Defined" class="DigNum (strict)"(error in=w482, "Precision"=w478) -> (error out=w481:errorcluster)  [unwired: 1 in, 1 out]
                      "CPT User Defined" <- w486
                      "PWP User Defined" <- w485
                      "Unit CPT User Defined" <- w484
                      "Unit PWP User Defined" <- w483
                    }
                    frame 1 {
                      n163 = property on="BPT User Defined" class="DigNum (strict)"(error in=w489, "Precision"=w488) -> (error out=w491:errorcluster)  [unwired: 1 in, 1 out]
                      n164 = property on="VC1 User Defined" class="DigNum (strict)"(error in=w491, "Precision"=w487) -> (error out=w490:errorcluster)  [unwired: 1 in, 1 out]
                      "BPT User Defined" <- w495
                      "VC1 User Defined" <- w494
                      "Unit BPT User Defined" <- w493
                      "Unit VC1 User Defined" <- w492
                    }
                    frame 2 {
                      n165 = property on="BPT2 User Defined" class="DigNum (strict)"(error in=w498, "Precision"=w497) -> (error out=w500:errorcluster)  [unwired: 1 in, 1 out]
                      n166 = property on="VC2 User Defined" class="DigNum (strict)"(error in=w500, "Precision"=w496) -> (error out=w499:errorcluster)  [unwired: 1 in, 1 out]
                      "BPT2 User Defined" <- w504
                      "VC2 User Defined" <- w503
                      "Unit BPT2 User Defined" <- w502
                      "Unit VC2 User Defined" <- w501
                    }
                    frame 3 {
                      n167 = property on="VL User Defined" class="DigNum (strict)"(error in=w507, "Precision"=w505) -> (error out=w509:errorcluster)  [unwired: 1 in, 1 out]
                      n168 = property on="VD User Defined" class="DigNum (strict)"(error in=w509, "Precision"=w506) -> (error out=w508:errorcluster)  [unwired: 1 in, 1 out]
                      "VL User Defined" <- w513
                      "VD User Defined" <- w512
                      "Unit VD User Defined" <- w510
                      "Unit VL User Defined" <- w511
                    }
                    frame 4 {
                      n169 = property on="HL User Defined" class="DigNum (strict)"(error in=w516, "Precision"=w515) -> (error out=w518:errorcluster)  [unwired: 1 in, 1 out]
                      n170 = property on="HD User Defined" class="DigNum (strict)"(error in=w518, "Precision"=w514) -> (error out=w517:errorcluster)  [unwired: 1 in, 1 out]
                      "HD User Defined" <- w521
                      "HL User Defined" <- w522
                      "Unit HD User Defined" <- w519
                      "Unit HL User Defined" <- w520
                    }
                  }
                }
              }
            }
          }
          frame "Delete" {
            n171 = Unbundle By Name(w558) -> ("Station Name"=w552:string)
            n172 = call "Station - Config File.vi"("Action"=enum16{"Write", "Read", "Read All", "Remove"}."Remove", "error in (no error)"=w553, "Station Name"=w552) -> ("error out"=w554:errorcluster)  [unwired: 7 in, 1 out]
            n173 = local write "Main Tab"(enum32{"Blank", "Edit"}."Blank" ("Main Tab")) -> ()
          }
          frame "Upload" {
            n174 = Unbundle By Name(w561) -> ("Station Name"=w579:string, "Table station"=w588:string[][], "EditRow"=w587:i32)
            n175 = property on="Test Type" class="Ring (strict)"(error in=w585) -> (error out=w582:errorcluster, "Strings []"=w584:string[])  [unwired: 1 in, 1 out]
            n176 = Index Array(array=w588, index (row)=w587, index (col)=2 ("disabled index (col)")) -> (element=w583:string)
            n177 = Search 1D Array(1D array=w584, element=w583) -> (index of element=w569:i32)  [unwired: 1 in]
            n178 = case shown="7" w569 {
              tunnel: [string[] [] string[] ["Test Type", "CPC Triaxial Shear", "BPC Triaxial Shear", "VLC Triaxial Shear", "Status"] string[] ["Test Type", "CPC Triaxial UU", "VLC Triaxial UU", "Status"] string[] ["Test Type", "VLC Shearbox", "HLC Shearbox", "Status"] string[] ["Test Type", "CPC Permeability", "BPC Permeability", "BPC2 Permeability", "Status"] string[] ["Test Type", "VLC Consolidation", "Status"] string[] ["Test Type", "CPC Saturation", "BPC Saturation", "Status"] string[] ["Test Type", "CPC User Defined", "BPC User Defined", "BPC2 User Defined", "VLC User Defined", "HLC User Defined", "Status"]] -> w568
              tunnel: w567 -> [_ w596 w599 w604 w609 w614 w619 w624]
              tunnel: [refnum<vi>[] [] w593 w598 w603 w608 w613 w618 w623] -> w566
              frame 0, Default {
              }
              frame 1 {
                n179 = Array Subset(array=w596, index=0, length=3) -> (w593:refnum<vi>[])
              }
              frame 2 {
                n180 = Array Subset(array=w599, index=3, length=2) -> (w598:refnum<vi>[])
              }
              frame 3 {
                n181 = Array Subset(array=w604, index=5, length=2) -> (w603:refnum<vi>[])
              }
              frame 4 {
                n182 = Array Subset(array=w609, index=7, length=3) -> (w608:refnum<vi>[])
              }
              frame 5 {
                n183 = Array Subset(array=w614, index=10, length=1) -> (w613:refnum<vi>[])
              }
              frame 6 {
                n184 = Array Subset(array=w619, index=11, length=2) -> (w618:refnum<vi>[])
              }
              frame 7 {
                n185 = Array Subset(array=w624, index=13, length=5) -> (w623:refnum<vi>[])
              }
            }
            n186 = property on="Test Type" class="Ring (strict)"(error in=w582, "Val(Sgnl)"=w569) -> (error out=w580:errorcluster)  [unwired: 1 in, 1 out]
            n187 = call "Station - Config File.vi"("Action"=enum16{"Write", "Read", "Read All", "Remove"}."Read", "error in (no error)"=w580, "Key Name"=w568, "Station Name"=w579) -> ("error out"=w571:errorcluster, "Value Out"=w578:T14)  [unwired: 6 in]
            n188 = Index Array(array=w578) -> (element=w577:T15)  [unwired: 1 in]
            n189 = Unbundle By Name(w577) -> ("Key Value"=w576:string[])
            n190 = Delete From Array(array=w576) -> (array with subset deleted=w575:string[])  [unwired: 2 in, 1 out]
            n191 = Delete From Array(array=w575, length=2, index=0) -> (deleted portion=w564:string[], array with subset deleted=w572:string[])
            n192 = global read "Global - Device.vi" "Device"() -> (w565:string[])
            n193 = Index Array(array=w564, index=1) -> (element=w560:string)
            "ID" <- w560
            n194 = for {
              tunnel: w572 -> [w633] mode=indexing
              tunnel: w565 -> [w634]
              shift-right: [w631] -> w570
              shift-left: w571 -> [w632]
              tunnel: w566 -> [w630] mode=indexing
              n195 = Search 1D Array(1D array=w634, element=w633) -> (index of element=w629:i32)  [unwired: 1 in]
              n196 = Increment(x=w629) -> (x+1=w628:i32)
              n197 = property class="Ring (strict)"(reference=w630, error in=w632, "Value"=w628) -> (error out=w631:errorcluster)  [unwired: 1 out]
            }
            n198 = Bundle By Name(cluster=w561, "Station ID"=w560) -> (w562:T5)
          }
          frame "save edit" {
            n199 = for {
              shift-right: [w647] -> w637
              shift-left: w641 -> [w648]
              tunnel: w640 -> [w646] mode=indexing
              tunnel: [w645] -> w642 mode=indexing
              n200 = property class="Ring (strict)"(reference=w646, error in=w648) -> (error out=w647:errorcluster, "RingText.Text"=w645:string)  [unwired: 1 out]
            }
            n201 = local read "Sub Tab"() -> (w639:T1)
            n202 = case shown="\"User Defined\"" w639 {
              tunnel: [string[] [] string[] ["Cell Pressure Control", "Back Pressure Control", "Vertical Load Control"] string[] ["Cell Pressure Control", "Vertical Load Control"] string[] ["Vertical Load Control", "Horizontal Load Control"] string[] ["Cell Pressure Control", "Back Pressure Control", "Back Pressure 2 Control"] string[] ["Vertical Load Control"] string[] ["Cell Pressure Control", "Back Pressure Control"] string[] ["Cell Pressure Control", "Back Pressure Control", "Back Pressure 2 Control", "Vertical Load Control", "Horizontal Load Control"]] -> w635
              tunnel: w642 -> [_ w654 w657 w662 w667 w672 w677 w682]
              tunnel: [string[] [] w651 w656 w661 w666 w671 w676 w681] -> w636
              frame "Please Select", Default {
              }
              frame "Triaxial Shear" {
                n203 = Array Subset(array=w654, index=0, length=3) -> (w651:string[])
              }
              frame "Triaxial UU" {
                n204 = Array Subset(array=w657, index=3, length=2) -> (w656:string[])
              }
              frame "Shearbox" {
                n205 = Array Subset(array=w662, index=5, length=2) -> (w661:string[])
              }
              frame "Permeability" {
                n206 = Array Subset(array=w667, index=7, length=3) -> (w666:string[])
              }
              frame "Consolidation" {
                n207 = Array Subset(array=w672, index=10, length=1) -> (w671:string[])
              }
              frame "Saturation" {
                n208 = Array Subset(array=w677, index=11, length=2) -> (w676:string[])
              }
              frame "User Defined" {
                n209 = Array Subset(array=w682, index=13, length=5) -> (w681:string[])
              }
            }
            "Device Name" <- w636
            "Key Name" <- w635
          }
          frame "Close" {
            n210 = control-ref of="This VI"() -> (w687:refnum<vi>)
            n211 = invoke class="VI" method="FP.Close"(reference=w687, error in=w691) -> (error out=w688:errorcluster)  [unwired: 1 in, 2 out]
          }
          frame "Exit" {
            n212 = control-ref of="This VI"() -> (w694:refnum<vi>)
            n213 = invoke class="VI" method="FP.Close"(reference=w694, error in=w692) -> (error out=w693:errorcluster)  [unwired: 1 in, 2 out]
          }
        }
      }
      frame Error {
        n214 = Unbundle By Name(w699) -> ("source"=w704:string)
        n215 = call <vilib>:"Clear Errors.vi"("error in (no error)"=w699) -> ("error out"=w701:errorcluster)  [unwired: 5 in, 1 out]
        n216 = Concatenate Strings("Station" ("string"), " - " ("string"), w704) -> (w702:string)
        n217 = call "General - Error Log eFGV.vi"("eFGV States"=eFGV_States."Write", "error in (no error)"=w701, "Error In"=w702) -> ("error out"=w700:errorcluster)  [unwired: 6 in, 2 out]
        n218 = Wait (ms)(milliseconds to wait=u32 100) -> ()  [unwired: 1 out]
      }
    }
  }
  "error out" <- w21
  n219 = disable-structure shown="Disabled" {
    frame Disabled {
      n220 = property on="Table" class="MCListbox (strict)"("ActiveCell"=T16 {"Row"=-2, "Column"=0} ("Active Cell:Active Cell"), "CellFontBold"=TRUE ("Active Cell:Cell Font:Bold")) -> ()  [unwired: 2 in, 2 out]
      n221 = for {
        N: 1000 -> [_]
        tunnel: T16 {"Row"=-2, "Column"=-2} ("Active Cell:Active Cell") -> [w722]
        i -> [w718]
        n222 = Bundle By Name(cluster=w722, "Row"=w718) -> (w723:T16)
        n223 = Quotient & Remainder(x=w718, y=2) -> (x-y*floor(x/y)=w716:i32)  [unwired: 1 out]
        n224 = Equal To 0?(x=w716) -> (x = 0?=w715:bool)
        n225 = Select(t=u32 16777225, s=w715, f=u32 16777238) -> (s? t:f=w719:u32)
        n226 = property on="Table" class="MCListbox (strict)"("ActiveCell"=w723, "Justify"=enum16{"Left", "Center", "Right"}."Center" ("Active Cell:Cell Justification"), "CellBG"=w719) -> ()  [unwired: 2 in, 2 out]
      }
    }
    frame Enabled {
    }
  }
